vi "Check RPC Engine Loop Stop Value.vi"(8 "error in (no error)":errorcluster) -> (0 "error out":errorcluster, 2 "stopped?":bool)   [LabVIEW 2017, in "JSONRPC Server.lvclass"]
uses:
  JSONRPC Server.lvclass
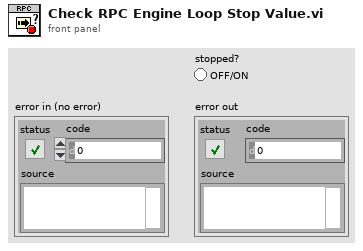
[diagram p1: front panel]
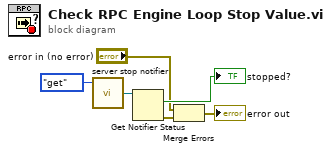
[diagram p0: block diagram]
diagram:
  n1 = call "server stop notifier.vi"("action"=enum16{"get", "set"}."get") -> ("notifier out"=w5:refnum<notifier>)  [unwired: 2 in]
  n2 = Get Notifier Status(notifier=w5) -> (current notification=→"stopped?":bool, error out=w2:errorcluster)  [unwired: 1 in, 3 out]
  n3 = Merge Errors("error in (no error)", w2) -> (→"error out":errorcluster)
